vi "Data Aquisition.vi"() -> ()   [LabVIEW 2018]
uses:
  <vilib>/Analysis/1siggen.llb/General Aperiodic Triangle.vi
  <instrlib>/RIGOL DG4000 Series/Public/Configure/Configure Standard Waveform(Square).vi
  <vilib>/Analysis/NI_AALBase.lvlib
  <instrlib>/RIGOL DG4000 Series/RIGOL DG4000 Series.lvlib
panel:
  in  "Tab Control":T1(tab)
  in  "Operator Name":string="ID-0"
  out "Simulated Data":dbl[][](graph)
  out "Numeric":i32
  in  "Department":string="EQD"
  in  "Start Samples":bool
  in  "bar code":string
  in  "Complete Samples":bool
  out "substring before match":string
  out "error out":errorcluster
  in  "error in (no error)":errorcluster
  in  "Duty Cycle (50 %)":dbl=50.0
  in  "Channel 1":bool=TRUE
  in  "Phase (0 Degree) 1":dbl format="%#_13g"
  in  "Phase (0 Degree) 2":dbl=180.0 format="%#_13g"
  in  "Channel  2":bool=TRUE
  in  "DC Offset (0.00 V)":dbl=1.65
  in  "Frequency (1000 Hz)":dbl=1.0
  in  "Amplitude (0.1 Vpp)":dbl=3.3
  in  "VISA resource name 2":refnum<visa-resource-name>
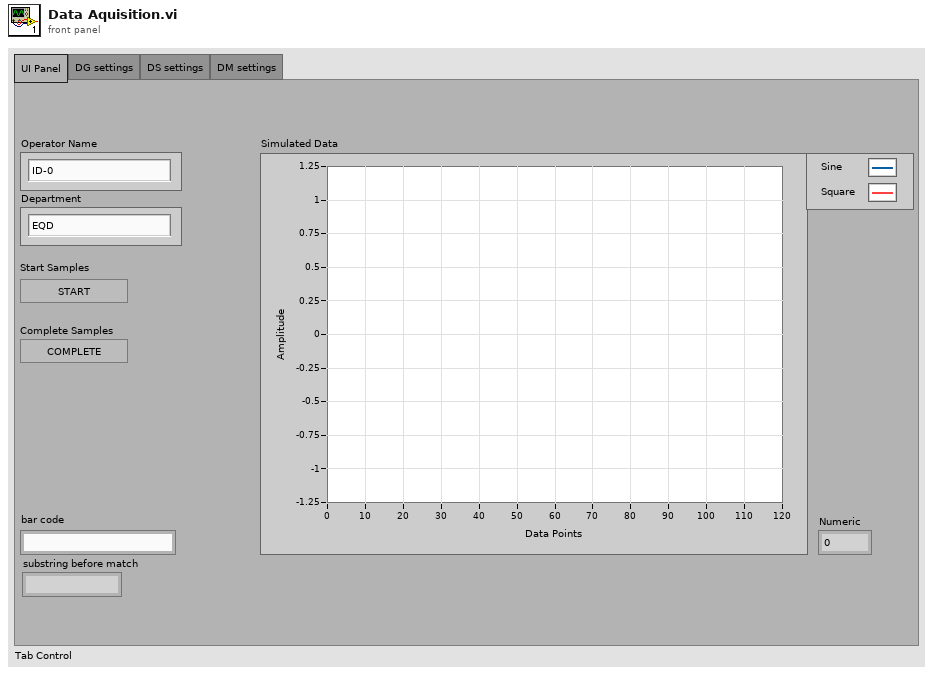
[diagram p1: front panel]
types:
  T1 = enum32{"UI Panel", "DG settings", "DS settings", "DM settings"}
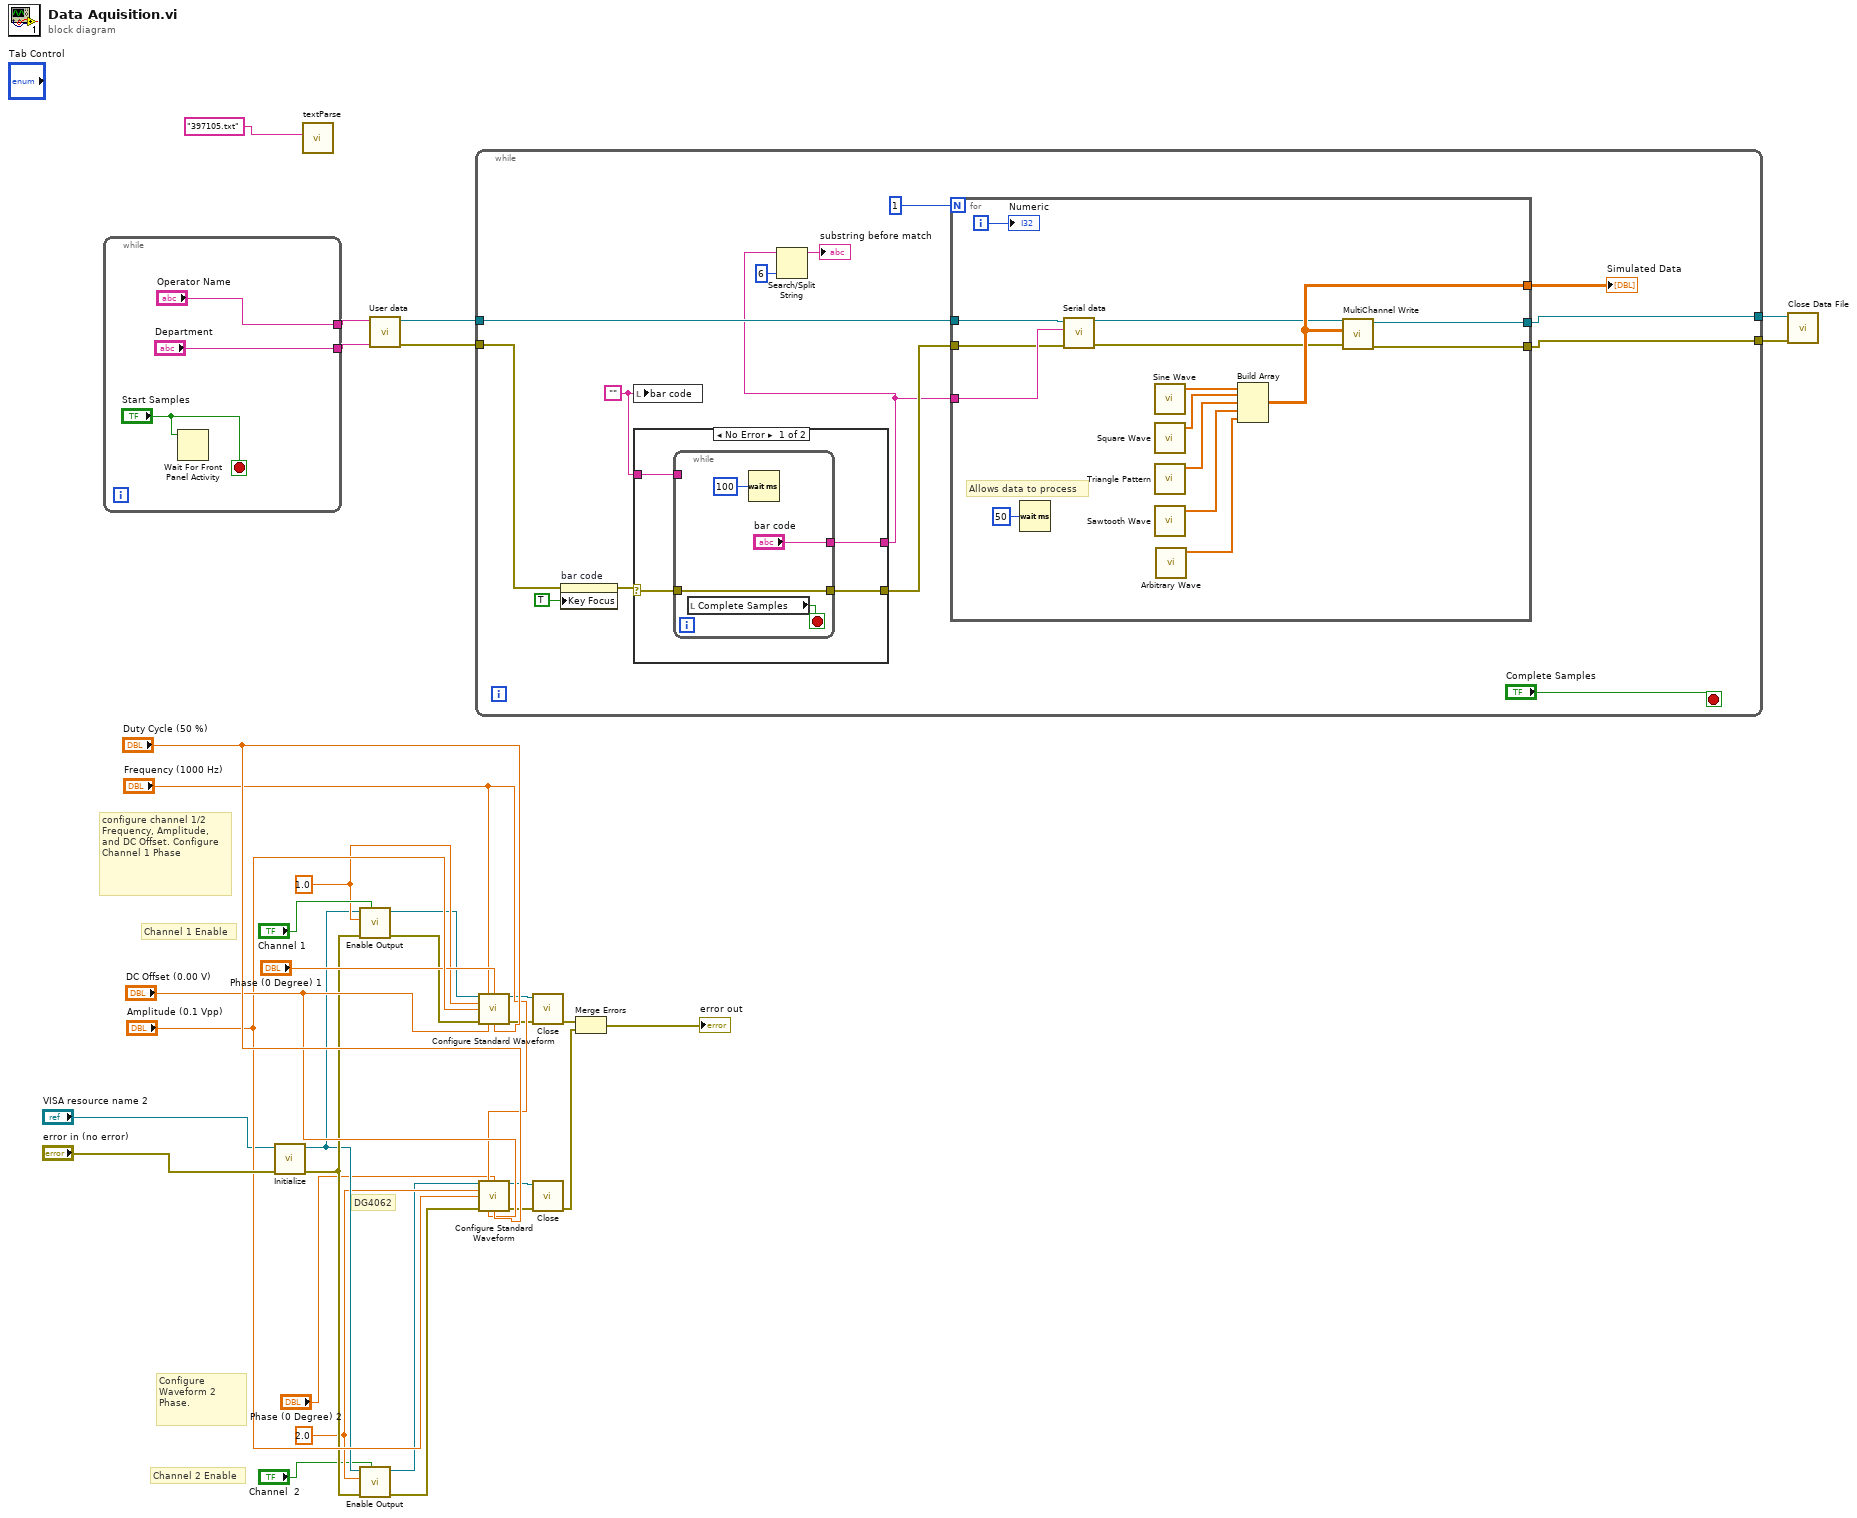
[diagram p0: block diagram]
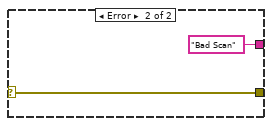
[diagram p2: hidden frame]
diagram:
  w19 = 1.0 ("Channel 2")
  w10 = 2.0 ("Channel")
  # "configure channel 1/2 Frequency, Amplitude, and DC Offset. Configure Channel 1 Phase"
  # "Channel 2 Enable"
  # "DG4062"
  # "Channel 1 Enable"
  # "Configure Waveform 2 Phase."
  n1 = while {
    tunnel: ["Operator Name"] -> w32
    tunnel: ["Department"] -> w30
    stop <- "Start Samples" stop-if-true
    n2 = Wait For Front Panel Activity(3:"Start Samples") -> ()  [unwired: 2 in, 1 out]
  }
  n3 = call <instrlib>:"Initialize.vi"("error in (no error)"="error in (no error)", "VISA resource name"="VISA resource name 2") -> ("error out"=w13:errorcluster, "VISA resource name out"=w12:refnum<visa-resource-name>)  [unwired: 3 in, 5 out]
  n4 = call "textParse.vi"("file name"="397105.txt" ("name or relative path")) -> ()  [unwired: 8 in, 3 out]
  n5 = call <instrlib>:"Enable Output.vi"("Enable Output (T: Enable)"="Channel 1", "error in (no error)"=w13, "Output Channel (1: Channel 1)"=w19, "VISA resource name"=w12) -> ("error out"=w15:errorcluster, "VISA resource name out"=w14:refnum<visa-resource-name>)  [unwired: 6 out]
  n6 = call <instrlib>:"Enable Output.vi"("Enable Output (T: Enable)"="Channel  2", "error in (no error)"=w13, "Output Channel (1: Channel 1)"=w10, "VISA resource name"=w12) -> ("error out"=w8:errorcluster, "VISA resource name out"=w7:refnum<visa-resource-name>)  [unwired: 6 out]
  n7 = call "User data.vi"("Operator Name"=w32, "Factory Name"=w30) -> ("refnum out"=w31:refnum<file>, "error out"=w4:errorcluster)  [unwired: 7 in]
  n8 = while {
    tunnel: w31 -> [w49]
    tunnel: w4 -> [w43]
    tunnel: [w41] -> w3
    tunnel: [w40] -> w2
    stop <- "Complete Samples" stop-if-true
    w46 = ""
    n9 = property on="bar code" class="Str"(error in=w43, "Key Focus"=TRUE) -> (error out=w45:errorcluster)  [unwired: 1 in, 1 out]
    n10 = local write "bar code"(w46) -> ()
    n11 = case shown="No Error" w45 {
      selector: w45 -> [w52 w59]
      tunnel: [w53 "Bad Scan" ("bar code")] -> w38
      tunnel: w46 -> [w51 _]
      tunnel: [w50 w59] -> w42
      frame No Error {
        n12 = while {
          tunnel: ["bar code"] -> w53
          tunnel: w52 -> [w55]
          tunnel: w51 -> [_]
          tunnel: [w55] -> w50
          stop <- w54 stop-if-true
          n13 = local read "Complete Samples"() -> (w54:bool)
          n14 = Wait (ms)(milliseconds to wait=u32 100) -> ()  [unwired: 1 out]
        }
      }
      frame Error {
      }
    }
    n15 = Search/Split String(string=w38, offset (0)=6) -> (substring before match=→"substring before match":string)  [unwired: 1 in, 2 out]
    n16 = for {
      N: 1 -> [_]
      tunnel: w49 -> [w62]
      tunnel: [w74] -> w41
      tunnel: [w73] -> w40
      tunnel: [w70] -> w48
      tunnel: w38 -> [w61]
      tunnel: w42 -> [w60]
      i -> [w69]
      # "Allows data to process"
      n17 = Wait (ms)(milliseconds to wait=u32 50) -> ()  [unwired: 1 out]
      n18 = call "Serial data.vi"("error in"=w60, "Serial Number"=w61, "refnum in"=w62) -> ("error out"=w63:errorcluster, "refnum out"=w64:refnum<file>)  [unwired: 7 in]
      n19 = call <vilib>:"Sine Wave.vi"() -> ("sine wave"=w71:dbl[])  [unwired: 5 in, 2 out]
      n20 = call <vilib>:"Square Wave.vi"() -> ("square wave"=w72:dbl[])  [unwired: 6 in, 2 out]
      n21 = call <vilib>:"Triangle Pattern.vi"() -> ("Triangle Pattern"=w67:dbl[])  [unwired: 10 in, 1 out]
      n22 = call <vilib>:"Sawtooth Wave.vi"() -> ("sawtooth wave"=w66:dbl[])  [unwired: 5 in, 2 out]
      n23 = call <vilib>:"Arbitrary Wave.vi"() -> ("arbitrary wave"=w65:dbl[])  [unwired: 7 in, 2 out]
      n24 = Build Array "Build Array"(w71, w72, w67, w66, w65) -> (w70:dbl[][])
      n25 = call "MultiChannel Write.vi"("Error In"=w63, "Data to Log"=w70, "File Refnum In"=w64) -> ("Error Out"=w74:errorcluster, "File Refnum Out"=w73:refnum<file>)  [unwired: 7 in]
      "Numeric" <- w69
    }
    "Simulated Data" <- w48
  }
  n26 = call-poly <instrlib>:"Configure Standard Waveform.vi"("VISA resource name"=w14, "Frequency (1000 Hz)"="Frequency (1000 Hz)", "Phase (0 Degree)"="Phase (0 Degree) 1", "Output Channel (1: Channel 1)"=w19, "Amplitude (5 Vpp)"="Amplitude (0.1 Vpp)", "error in (no error)"=w15, "Offset (0)"="DC Offset (0.00 V)", "Duty Cycle (50 %)"="Duty Cycle (50 %)") -> ("VISA resource name out"=w17:refnum<visa-resource-name>, "error out"=w18:errorcluster)  [unwired: 1 in, 5 out]
  n27 = call-poly <instrlib>:"Configure Standard Waveform.vi"("VISA resource name"=w7, "Frequency (1000 Hz)"="Frequency (1000 Hz)", "Phase (0 Degree)"="Phase (0 Degree) 2", "Output Channel (1: Channel 1)"=w10, "Amplitude (5 Vpp)"="Amplitude (0.1 Vpp)", "error in (no error)"=w8, "Offset (0)"="DC Offset (0.00 V)", "Duty Cycle (50 %)"="Duty Cycle (50 %)") -> ("VISA resource name out"=w16:refnum<visa-resource-name>, "error out"=w9:errorcluster)  [unwired: 1 in, 5 out]
  n28 = call <instrlib>:"Close.vi"("error in (no error)"=w18, "VISA resource name"=w17) -> ("error out"=w27:errorcluster)  [unwired: 9 out]
  n29 = call <instrlib>:"Close.vi"("error in (no error)"=w9, "VISA resource name"=w16) -> ("error out"=w28:errorcluster)  [unwired: 9 out]
  n30 = Merge Errors(w27, w28) -> (→"error out":errorcluster)
  n31 = call "Close Data File.vi"("error in"=w3, "File Refnum In"=w2) -> ()  [unwired: 9 in, 1 out]
